vi "TwGetBufTimeFromH5.vi"(2 "writeIndex":i32, 3 "bufIndex":i32, 4 "filename":string, 5 "error in (no error)":errorcluster) -> (0 "bufTime":dbl, 1 "error out":errorcluster)   [LabVIEW 2009]
uses:
  TwH5Dll.dll
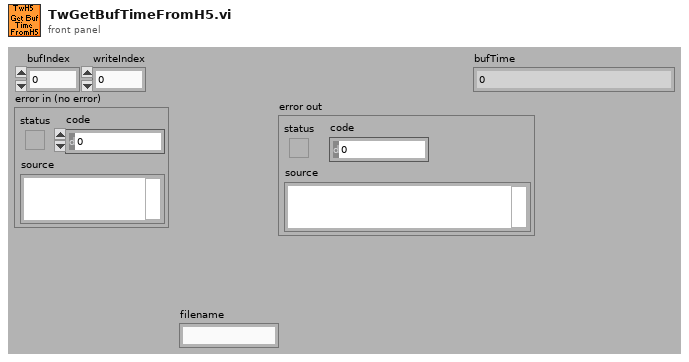
[diagram p1: front panel]
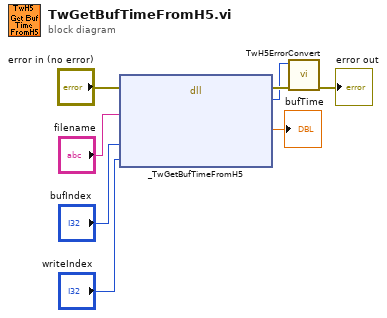
[diagram p0: block diagram]
diagram:
  n1 = dll-call lib="C:/src/85_TofDaq_current/DllWrappers/LabView/TwH5Dll/TwH5Dll.dll" fn="_TwGetBufTimeFromH5"(error in="error in (no error)", "filename"="filename", "bufIndex"="bufIndex", "writeIndex"="writeIndex") -> (error out=w7:errorcluster, "TwRetVal"=w6:i32, "bufTime"=→"bufTime":dbl)  [unwired: 5 in, 2 out]
  n2 = call "TwH5ErrorConvert.vi"("error in (no error)"=w7, "error code"=w6) -> ("error out"=→"error out":errorcluster)  [unwired: 9 out]
